vi "graph configuration.vi"(3 "extras?":bool, 4 "width":u8, 5 "style":u8, 6 "BG":u32(colorbox)=16448250, 7 "scale":dbl format="%#_13g", 8 "line color":u32(colorbox)=16448250, 9 "multiplicator":i32=1, 10 "loops":i32=1, 11 "graph":refnum<vi>) -> ()   [LabVIEW 2014]
uses:
  <vilib>/Utility/miscctls.llb/LVMajorAndMinorColorsTypeDef.ctl
  <vilib>/Utility/miscctls.llb/LVRectTypeDef.ctl
panel:
  in  "graph":cluster{"x":dbl[], "y":dbl[]}[](graph)
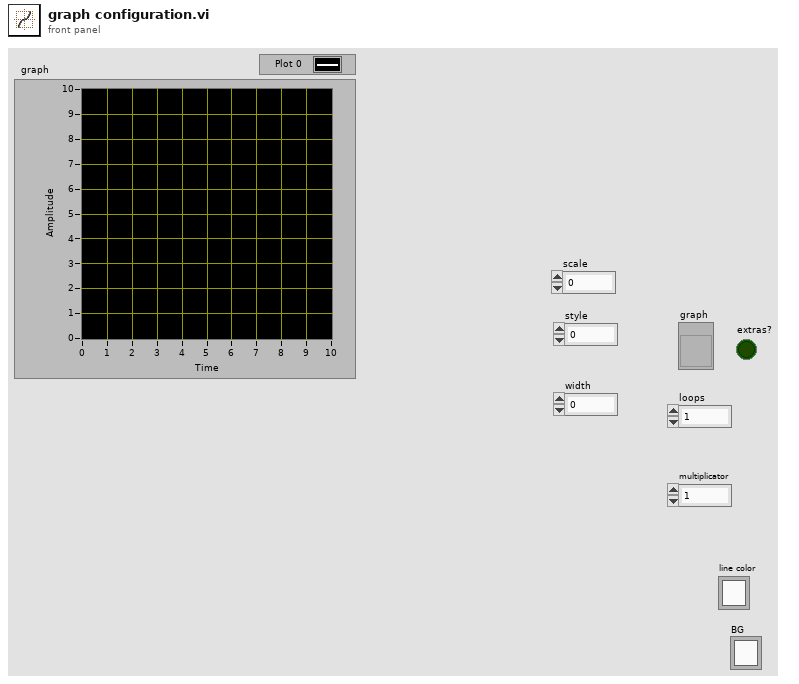
[diagram p1: front panel]
types:
  T1 = typedef "LVRectTypeDef.ctl" = cluster{"Left":i16, "Top":i16, "Right":i16, "Bottom":i16}
  T2 = typedef "LVMajorAndMinorColorsTypeDef.ctl" = cluster{"Major Color":u32, "Minor Color":u32}
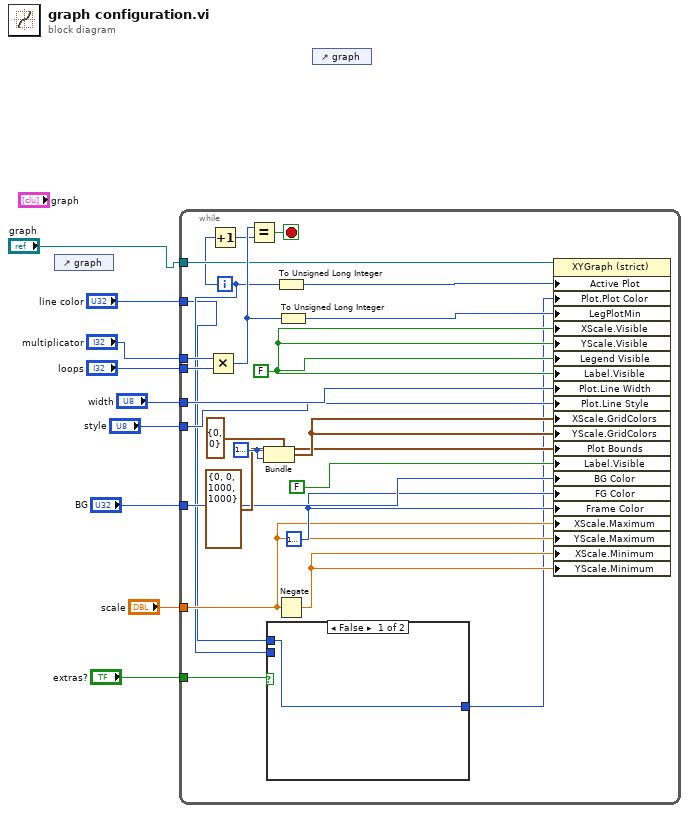
[diagram p0: block diagram]
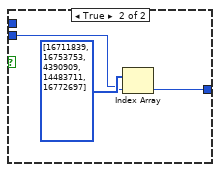
[diagram p2: hidden frame]
diagram:
  n1 = control-ref of="graph"() -> ()  [unwired: 1 out]
  n2 = while {
    tunnel: "loops" -> [w28]
    tunnel: "graph" -> [w27]
    tunnel: "line color" -> [w11]
    tunnel: "multiplicator" -> [w26]
    tunnel: "BG" -> [w20]
    tunnel: "scale" -> [w17]
    tunnel: "width" -> [w16]
    tunnel: "style" -> [w15]
    tunnel: "extras?" -> [w13]
    i -> [w12]
    stop <- w33 stop-if-true
    w19 = u32 16777216
    w25 = u32 16777216
    w14 = FALSE ("Label.Visible")
    n3 = Multiply(x=w26, y=w28) -> (x*y=w32:i32)
    n4 = Increment(x=w12) -> (x+1=w30:i32)
    n5 = Equal?(x=w32, y=w30) -> (x = y?=w33:bool)
    n6 = Bundle(cluster=T2 {"Major Color"=0, "Minor Color"=0} ("X Scale.Grid Colors"), "Major Color"=w25, "Minor Color"=w25) -> (w23:T2)
    n7 = case shown="False" w13 {
      tunnel: w12 -> [_ w36]
      tunnel: [w34 w35] -> w10
      tunnel: w11 -> [w34 _]
      frame False {
      }
      frame True {
        n8 = Index Array(array=u32[] [16711839, 16753753, 4390909, 14483711, 16772697], index=w36) -> (element=w35:u32)
      }
    }
    n9 = To Unsigned Long Integer(number=w12) -> (unsigned 32bit integer=w29:u32)
    n10 = Negate(x=w17) -> (-x=w18:dbl)
    n11 = To Unsigned Long Integer(number=w32) -> (unsigned 32bit integer=w31:u32)
    n12 = property on="Property Node" class="XYGraph (strict)"(reference=w27, "Active Plot"=w29, "Plot.Plot Color"=w10, "LegPlotMin"=w31, "XScale.Visible"=w14, "YScale.Visible"=w14, "Legend Visible"=w14, "Label.Visible"=w14, "Plot.Line Width"=w16, "Plot.Line Style"=w15, "XScale.GridColors"=w23, "YScale.GridColors"=w23, "Plot Bounds"=T1 {"Left"=0, "Top"=0, "Right"=1000, "Bottom"=1000} ("Plot Area Bounds"), "Label.Visible"=FALSE, "BG Color"=w20, "FG Color"=w19, "Frame Color"=w19, "XScale.Maximum"=w17, "YScale.Maximum"=w17, "XScale.Minimum"=w18, "YScale.Minimum"=w18) -> ()  [unwired: 1 in, 2 out]
  }
  n13 = control-ref of="graph"() -> ()  [unwired: 1 out]
